vi "Complimentry Filter.vi"(7 "Filter Coefficient a":dbl, 8 "dt (ms)":u32, 10 "Gyro (degrees/second)":dbl, 11 "Accelerometer (degrees)":dbl) -> (2 "timeConstant":dbl, 3 "Filtered":dbl)   [LabVIEW 2014]
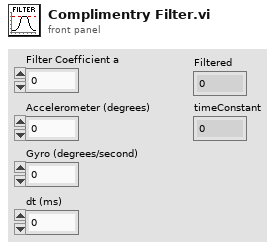
[diagram p1: front panel]
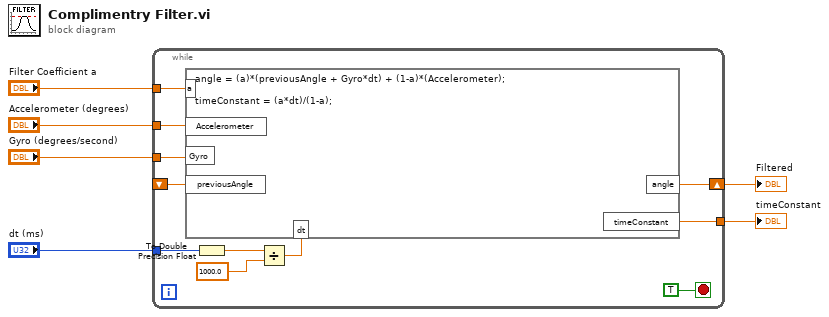
[diagram p0: block diagram]
diagram:
  n1 = while {
    shift-right: [w12] -> w4
    shift-left: _ -> [w9]
    tunnel: "Accelerometer (degrees)" -> [w8]
    tunnel: "Gyro (degrees/second)" -> [w10]
    tunnel: "Filter Coefficient a" -> [w13]
    tunnel: "dt (ms)" -> [w14]
    tunnel: [w7] -> w1
    stop <- TRUE stop-if-true
    n2 = To Double Precision Float(number=w14) -> (double precision float=w15:dbl)
    n3 = Divide(x=w15, y=1000.0 ("x")) -> (x/y=w11:dbl)
    n4 = formula code="angle = (a)*(previousAngle + Gyro*dt) + (1-a)*(Accelerometer);\n\ntimeConstant = (a*dt)/(1-a);"("a"=w13, "previousAngle"=w9, "dt"=w11, "Accelerometer"=w8, "Gyro"=w10) -> ("angle"=w12:dbl, "timeConstant"=w7:dbl)
  }
  "Filtered" <- w4
  "timeConstant" <- w1
